vi "inference_23Q3.vi"() -> ()   [LabVIEW 2023]
panel:
  out "appended path":path
  out "result string":string
  out "return value":string
  out "string":string
  out "Application Directory":path
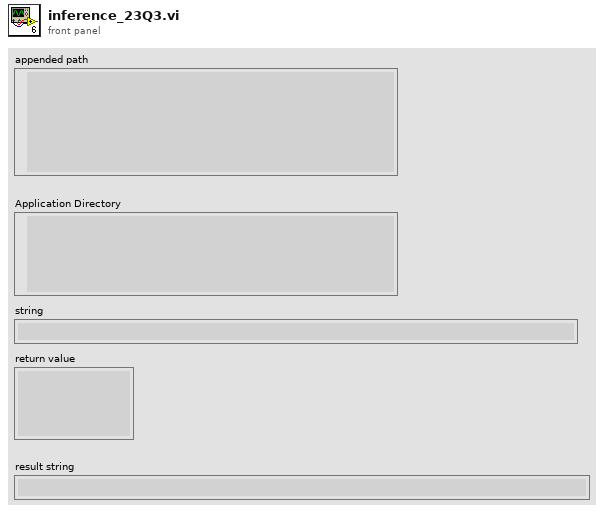
[diagram p1: front panel]
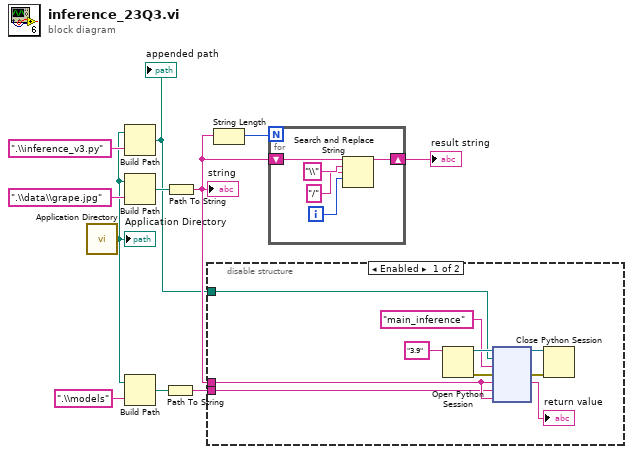
[diagram p0: block diagram]
diagram:
  n1 = call <vilib>:"Application Directory.vi"() -> ("Application Directory"=w2:path)
  "Application Directory" <- w2
  n2 = Build Path(base path=w2, name or relative path=".\\inference_v3.py") -> (appended path=w1:path)
  "appended path" <- w1
  n3 = Build Path(base path=w2, name or relative path=".\\data\\grape.jpg") -> (appended path=w10:path)
  n4 = Build Path(base path=w2, name or relative path=".\\models") -> (appended path=w8:path)
  n5 = Path To String(path=w8) -> (string=w7:string)
  n6 = Path To String(path=w10) -> (string=w5:string)
  "string" <- w5
  n7 = disable-structure shown="Enabled" {
    disable-tunnel: w5 -> [w15 _]
    disable-tunnel: w7 -> [w14 _]
    disable-tunnel: w1 -> [w12 _]
    frame Enabled {
      n8 = Open Python Session(python version="3.9" ("Python version")) -> (session out=w21:refnum<k35>, error out=w20:errorcluster)  [unwired: 2 in]
      n9 = node(w21, w12, "main_inference" ("function name"), w20, w15, w14, w15) -> (w19:refnum<k35>, w18:errorcluster, →"return value":string)  [unwired: 2 in, 2 out]
      n10 = Close Python Session(session in=w19, error in=w18) -> ()  [unwired: 1 out]
    }
    frame Disabled {
    }
  }
  n11 = String Length(string=w5) -> (length=w6:i32)
  n12 = for {
    N: w6 -> [_]
    shift-right: [w22] -> w4
    shift-left: w5 -> [w25]
    i -> [w23]
    n13 = Search and Replace String(input string=w25, search string="\\", replace string="/" ("replace string (\"\")"), offset=w23) -> (result string=w22:string)  [unwired: 4 in, 3 out]
  }
  "result string" <- w4
